vi "ReadExcel.vi"(8 "error in":errorcluster caption="错误输入（无错误）", 11 "template":path caption="模板（空）") -> (0 "error out":errorcluster caption="错误输出", 3 "data":string[][](array[string]))   [LabVIEW 2013]
uses:
  <vilib>/Utility/NIReport.llb/NI_report.lvclass
  <vilib>/addons/_office/excel.llb/Excel Get Data ([str]).vi
  <vilib>/addons/_office/NI_ReportGenerationToolkit.lvlib
  <vilib>/Utility/NIReport.llb/Excel/NI_Excel.lvclass
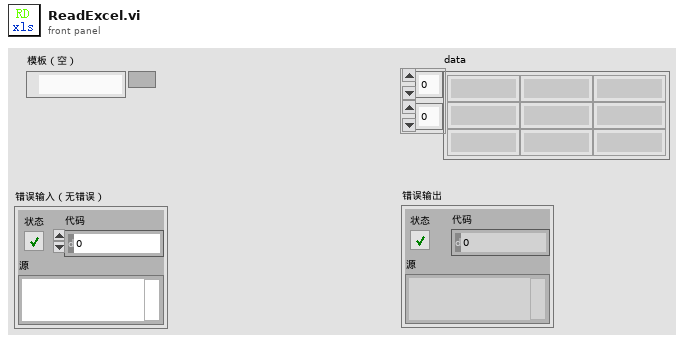
[diagram p1: front panel]
types:
  T1 = enum16{"maximized", "minimized", "normal", "no change"}
  T2 = enum16{"Standard Report", "HTML", "Word", "Excel"}
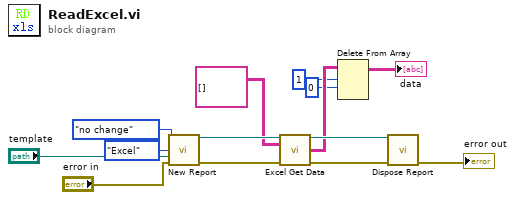
[diagram p0: block diagram]
diagram:
  n1 = call <vilib>:"New Report.vi"("window state (normal)"=T1."no change", "report type"=T2."Excel", "template (empty)"="template", "error in (no error)"="error in") -> ("report out"=w11:refnum<class "NI_report.lvclass">, "error out"=w10:errorcluster)  [unwired: 10 in]
  n2 = call-poly <vilib>:"Excel Get Data.vi"("report in"=w11, "data type"=string[][] [], "error in (no error)"=w10) -> ("report out"=w8:refnum<class "NI_report.lvclass">, "data"=w4:string[][], "error out"=w7:errorcluster)  [unwired: 10 in]
  n3 = Delete From Array(array=w4, length=1 ("长度"), index (row)=0 ("索引 (行)")) -> (array with subset deleted=→"data":string[][])  [unwired: 1 in, 1 out]
  n4 = call-dynamic "Dispose Report.vi"("report in"=w8, "error in (no error)"=w7) -> ("error out"=→"error out":errorcluster)  [unwired: 13 in]
